vi "globals.vi"() -> ()   [LabVIEW 2016, in "ds402mgr_Helper.lvlib"]
uses:
  ds402mgr_Helper.lvlib
panel:
  in  "ECAT position address":string="user.CD.ECAT Slave #"
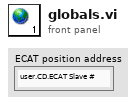
[diagram p1: front panel]
diagram:
